vi "find_MFTObject_by_name.vi"(8 "error in (no error)":errorcluster, 10 "MFT name":string, 11 "MFTObjects in":refnum<class "MagFieldTable.lvclass">[](array[class])) -> (0 "error out":errorcluster, 1 "index of found":i32, 2 "found AnalyisObject":refnum<class "MagFieldTable.lvclass">, 3 "MFTObjects out":refnum<class "MagFieldTable.lvclass">[](array[class]))   [LabVIEW 2018]
doc: "finds the isotope in the magfield tables"
uses:
  Classes/MagFieldTable/MagFieldTable.lvclass
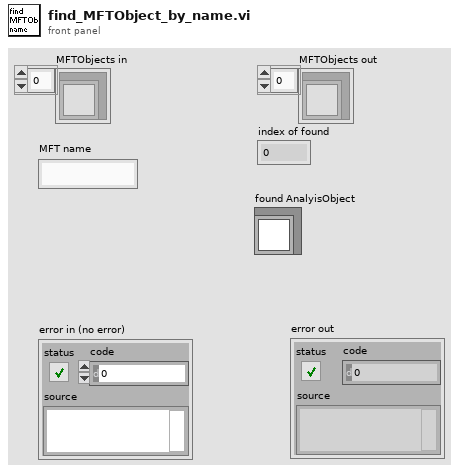
[diagram p1: front panel]
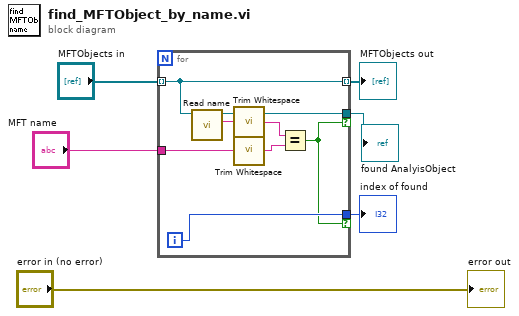
[diagram p0: block diagram]
diagram:
  n1 = for {
    tunnel: "MFTObjects in" -> [w9] mode=indexing
    tunnel: "MFT name" -> [w13]
    tunnel: [w10] -> w2 if=w7
    tunnel: [w9] -> w4 mode=indexing
    tunnel: [w8] -> w3 if=w7
    i -> [w8]
    n2 = call-dynamic "Read name.vi"("MagFieldTable in"=w9) -> ("name"=w14:string, "MagFieldTable out"=w10:refnum<class "MagFieldTable.lvclass">)  [unwired: 8 in, 1 out]
    n3 = call <vilib>:"Trim Whitespace.vi"("string"=w14) -> ("trimmed string"=w12:string)  [unwired: 1 in]
    n4 = call <vilib>:"Trim Whitespace.vi"("string"=w13) -> ("trimmed string"=w11:string)  [unwired: 1 in]
    n5 = Equal?(x=w12, y=w11) -> (x = y?=w7:bool)
  }
  "found AnalyisObject" <- w2
  "MFTObjects out" <- w4
  "index of found" <- w3
  "error out" <- "error in (no error)"
